vi "PID Internals_V.vi"(0 "Run PI?":bool, 1 "PIcluster":cluster{"SlewRate":dbl, "Kp":dbl, "Ki":dbl}, 2 "FFcluster":cluster{"FF_m":dbl, "FF_b":dbl}, 3 "LimitCluster":T1, 5 "SP":dbl, 7 "Error":dbl, 11 "RevCtrlZero":bool, 13 "Indirect FF":bool) -> (4 "PreSlew":dbl, 8 "Output":dbl)   [LabVIEW 2013]
uses:
  <vilib>/addons/control/pid/pid.llb/PID Output Rate Limiter (DBL).vi
  <vilib>/addons/control/pid/NI_PID_pid.lvlib
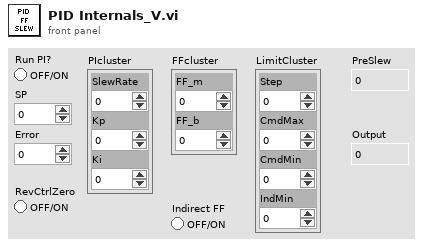
[diagram p1: front panel]
types:
  T1 = cluster{"Step":dbl, "CmdMax":dbl, "CmdMin":dbl, "IndMin":dbl}
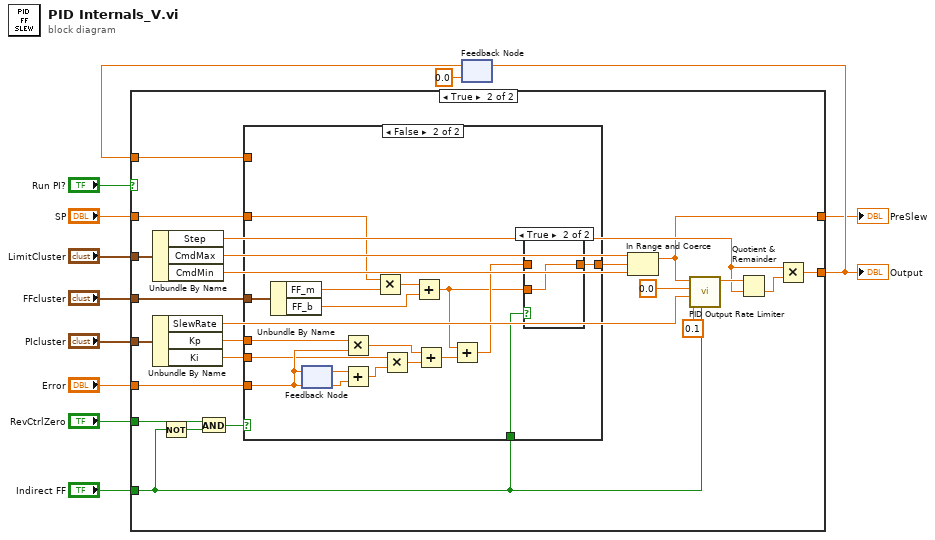
[diagram p0: block diagram]
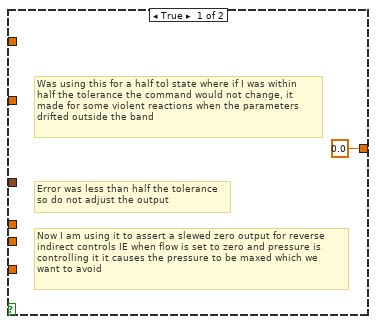
[diagram p3: hidden frame]
diagram:
  n1 = feedback #1(0.0 ("SP")) -> (w4:dbl)
  n2 = case shown="True" "Run PI?" {
    tunnel: [w13 w24] -> w5
    tunnel: "SP" -> [w13 w36]
    tunnel: "Error" -> [_ w35]
    tunnel: "FFcluster" -> [_ w34]
    tunnel: "PIcluster" -> [_ w31]
    tunnel: "LimitCluster" -> [_ w32]
    tunnel: "RevCtrlZero" -> [_ w19]
    tunnel: w4 -> [_ w33]
    tunnel: [w13 w16] -> w2
    tunnel: "Indirect FF" -> [_ w15]
    frame False {
    }
    frame True {
      n3 = Unbundle By Name(w32) -> ("Step"=w25:dbl, "CmdMax"=w22:dbl, "CmdMin"=w21:dbl)
      n4 = Unbundle By Name(w31) -> ("SlewRate"=w26:dbl, "Kp"=w30:dbl, "Ki"=w29:dbl)
      n5 = Not(x=w15) -> (.not. x?=w18:bool)
      n6 = And(x=w19, y=w18) -> (x .and. y?=w17:bool)
      n7 = case shown="False" w17 {
        tunnel: w36 -> [_ w52]
        tunnel: w35 -> [_ w50]
        tunnel: w34 -> [_ w46]
        tunnel: w33 -> [_ _]
        tunnel: w30 -> [_ w43]
        tunnel: w29 -> [_ w42]
        tunnel: [0.0 ("CmdMax") w39] -> w23
        tunnel: w15 -> [_ w41]
        frame True {
          # "Now I am using it to assert a slewed zero output for reverse\nindirect controls IE when flow is set to zero and pressure is\ncontrolling it it causes the pressure to be maxed which we\nwant to avoid"
          # "Was using this for a half tol state where if I was within\nhalf the tolerance the command would not change, it\nmade for some violent reactions when the parameters\ndrifted outside the band"
          # "Error was less than half the tolerance\nso do not adjust the output"
        }
        frame False {
          n8 = Unbundle By Name(w46) -> ("FF_m"=w45:dbl, "FF_b"=w44:dbl)
          n9 = feedback #2(w50) -> (w51:dbl)
          n10 = feedback-in #2(w50) -> ()
          n11 = Multiply(x=w43, y=w50) -> (x*y=w48:dbl)
          n12 = Add(x=w51, y=w50) -> (x+y=w47:dbl)
          n13 = Multiply(x=w52, y=w45) -> (x*y=w54:dbl)
          n14 = Multiply(x=w42, y=w47) -> (x*y=w49:dbl)
          n15 = Add(x=w54, y=w44) -> (x+y=w38:dbl)
          n16 = Add(x=w48, y=w49) -> (x+y=w53:dbl)
          n17 = Add(x=w38, y=w53) -> (x+y=w40:dbl)
          n18 = case shown="True" w41 {
            tunnel: w40 -> [w55 _]
            tunnel: [w55 w56] -> w39
            tunnel: w38 -> [_ w56]
            frame False {
            }
            frame True {
            }
          }
        }
      }
      n19 = In Range and Coerce(upper limit=w22, x=w23, lower limit=w21) -> (coerced(x)=w16:dbl)  [unwired: 1 out]
      n20 = call-poly <vilib>:"PID Output Rate Limiter.vi"("reinitialize? (F)"=w15, "dt (s)"=0.1, "output rate (EGU/min)"=w26, "initial output"=0.0, "input (controller output)"=w16) -> ("output"=w28:dbl)  [unwired: 3 in, 1 out]
      n21 = Quotient & Remainder(x=w28, y=w25) -> (floor(x/y)=w27:dbl)  [unwired: 1 out]
      n22 = Multiply(x=w25, y=w27) -> (x*y=w24:dbl)
    }
  }
  "Output" <- w5
  "PreSlew" <- w2
  n23 = feedback-in #1(w5) -> ()
